vi "Hex字令变换.vi"(2 "error in (no error)":errorcluster caption="错误输入（无错误）", 3 "数值":dbl) -> (0 "error out":errorcluster caption="错误输出", 1 "Hex指令":u32[](array[numeric]) format="%.0x")   [LabVIEW 2015, in "MSP6715.lvlib"]
uses:
  MSP6715.lvlib
panel:
  out "floor(x/y)":u32 format="%.0x"
  out "x-y*floor(x/y)":u32 format="%.0x"
  out "y":u32 format="%.0x"
  out "添加的数组":u32[](array[numeric]) format="%.0x"
  out "数组 2":u32[](array[numeric]) format="%.0x"
  out "数组":string[](array[string])
  out "字符串":string
  out "十六进制整型字符串":string
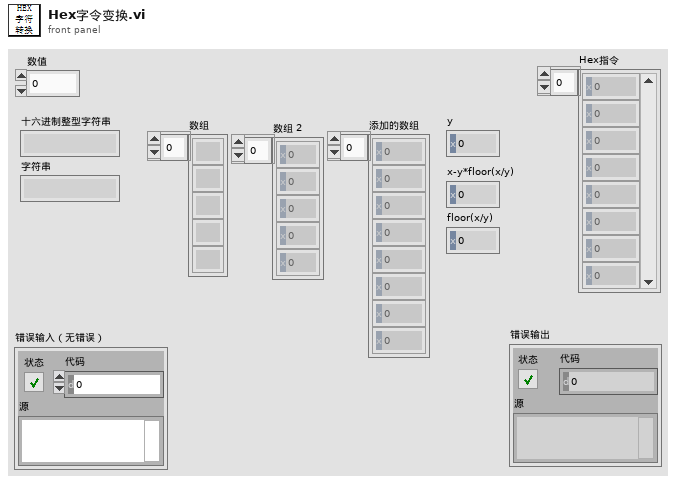
[diagram p1: front panel]
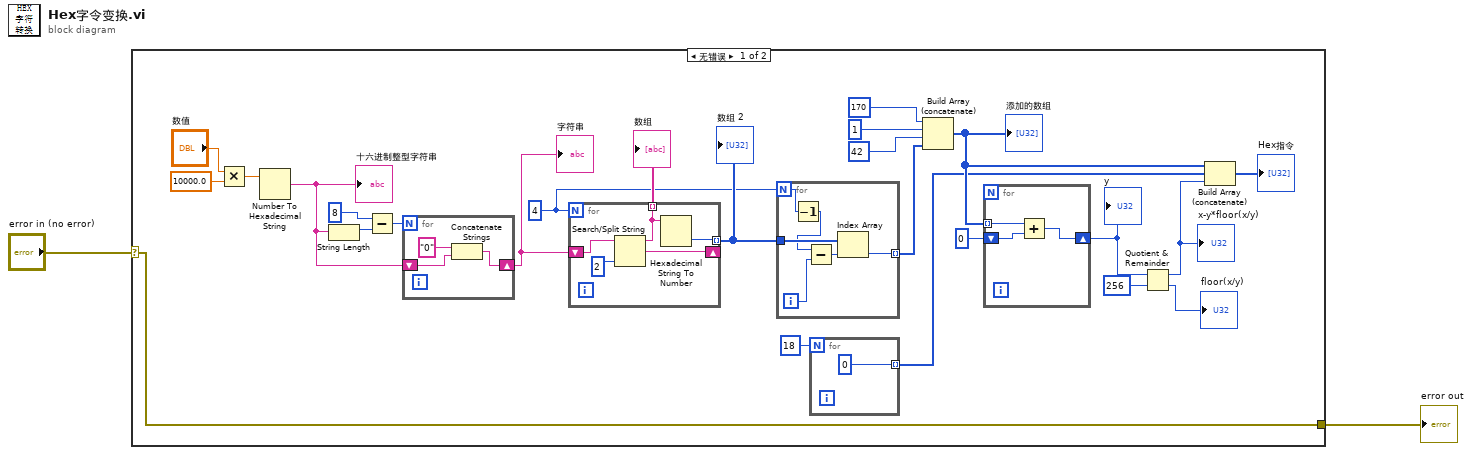
[diagram p0: block diagram]
diagram:
  n1 = case shown="无错误" "error in (no error)" {
    selector: "error in (no error)" -> [w3 w46]
    tunnel: [w3 w46] -> w1
    frame No Error {
      w14 = 4
      n2 = Multiply(x="数值", y=10000.0) -> (x*y=w25:dbl)
      n3 = Number To Hexadecimal String(2:w25) -> (0:w21:string)  [unwired: 1 in]
      "十六进制整型字符串" <- w21
      n4 = String Length(string=w21) -> (length=w23:i32)
      n5 = Subtract(x=8, y=w23) -> (x-y=w22:i32)
      n6 = for {
        N: w22 -> [_]
        shift-right: [w43] -> w20
        shift-left: w21 -> [w45]
        n7 = Concatenate Strings("0", w45) -> (w43:string)
      }
      "字符串" <- w20
      n8 = for {
        N: w14 -> [_]
        shift-right: [w40] -> _
        shift-left: w20 -> [w42]
        tunnel: [w39] -> w15 mode=indexing
        tunnel: [w38] -> w19 mode=indexing
        n9 = Search/Split String(string=w42, offset (0)=2 ("长度（剩余）")) -> (substring before match=w38:string, match + rest of string=w40:string)  [unwired: 1 in, 1 out]
        n10 = Hexadecimal String To Number(string=w38) -> (number=w39:u32)  [unwired: 2 in, 1 out]
      }
      "数组" <- w19
      "数组 2" <- w15
      n11 = for {
        N: w14 -> [w33]
        tunnel: w15 -> [w37]
        tunnel: [w34] -> w13 mode=indexing
        i -> [w35]
        n12 = Decrement(x=w33) -> (x-1=w32:i32)
        n13 = Subtract(x=w32, y=w35) -> (x-y=w36:i32)
        n14 = Index Array(array=w37, index=w36) -> (element=w34:u32)
      }
      n15 = for {
        N: 18 -> [_]
        tunnel: [0] -> w6 mode=indexing
      }
      n16 = Build Array (concatenate)(170, 1, 42, w13) -> (w7:u32[])
      "添加的数组" <- w7
      n17 = for {
        tunnel: w7 -> [w30] mode=indexing
        shift-right: [w28] -> w10
        shift-left: u32 0 ("y") -> [w29]
        n18 = Add(x=w30, y=w29) -> (x+y=w28:u32)
      }
      "y" <- w10
      n19 = Quotient & Remainder(x=w10, y=u32 256) -> (x-y*floor(x/y)=w5:u32, floor(x/y)=→"floor(x/y)":u32)
      "x-y*floor(x/y)" <- w5
      n20 = Build Array (concatenate)(w7, w6, w5) -> (→"Hex指令":u32[])
    }
    frame Error {
    }
  }
  "error out" <- w1
